vi "Write to Hardware.vi"(8 "error in":errorcluster, 9 "trigger values":dbl[](array[numeric]), 10 "Values in":dbl[](array[numeric]), 11 "Ballard ARINC-429 Tx Acyclic execution unit in":refnum<class "Tx Acyclic Labels Execution Unit.lvclass">) -> (0 "error out":errorcluster, 1 "trigger values out":dbl[](array[numeric]), 2 "Values out":dbl[](array[numeric]), 3 "Ballard ARINC-429 Tx Acyclic execution unit out":refnum<class "Tx Acyclic Labels Execution Unit.lvclass">)   [LabVIEW 2020, in "Ballard ARINC 429 Engine.lvlib" / "Implementation.lvlib" / "Tx Acyclic Labels Execution Unit.lvclass"]
uses:
  Tx Acyclic Labels Execution Unit.lvclass
  <instrlib>/BTI429Lib/BTI429LV.lvlib
  <instrlib>/BTI429Lib/Private/Tx/Data/Transmit Message Dynamic.vi
  Custom Device/Custom Device.lvlib
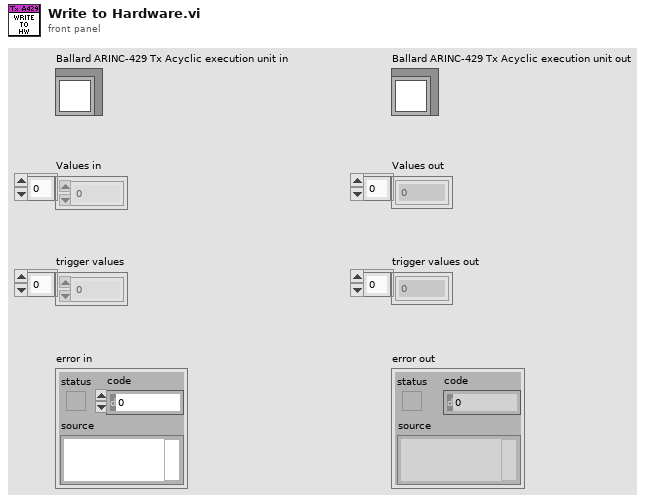
[diagram p1: front panel]
types:
  T1 = typedef "RT Hardware Channel Settings.ctl" = cluster{"channel #":u16, "channel handle":u64, "labels settings for RT":T2[]}
  T2 = typedef "RT Label Settings.ctl" = cluster{"Name":string, "xmlName":string, "label":T3, "transfer period":u32, "SDI_Enabled":bool, "SDI":u8, "parameter driver data":T4, "transfer type":T8, "has timestamp?":bool, "Label Disable/Trigger Channel Reference":T7, "Message Handle":u64, "Initialized?":bool, "Word Initial Raw Value":u32, "Label Timestamp Channel Data Reference":T9, "disabled":bool}
  T3 = typedef "Label.ctl" = u8
  T4 = typedef "RT Parameters.ctl" = cluster{"parameter definitions":T5[], "Tx parameter refs":T7[]}
  T5 = typedef "Parameter Definition.ctl" = cluster{"start index":i32, "size":i32, "encoding":T6, "signed":bool, "scale multiplier":dbl, "scale offset":dbl}
  T6 = typedef "Encoding and Decoding.lvlib/Encoding.ctl" = enum16{"BNR", "BCD", "Discrete"}
  T7 = typedef "Custom Device API.lvlib/Custom Device Item Ref.ctl" = u64
  T8 = typedef "Transfer Type.ctl" = enum16{"Scheduled", "Acyclic", "Block", "Strobe"}
  T9 = typedef "Custom Device API.lvlib/Data Reference.ctl" = i32
  T10 = typedef "Map of Values Indexes to Channel and Label Indexes.ctl" = map{i32, cluster{"channel index":i32, "label index":i32, "group values start index":i32, "values in group":i32}}
  T11 = cluster{"channel index":i32, "label index":i32, "group values start index":i32, "values in group":i32}
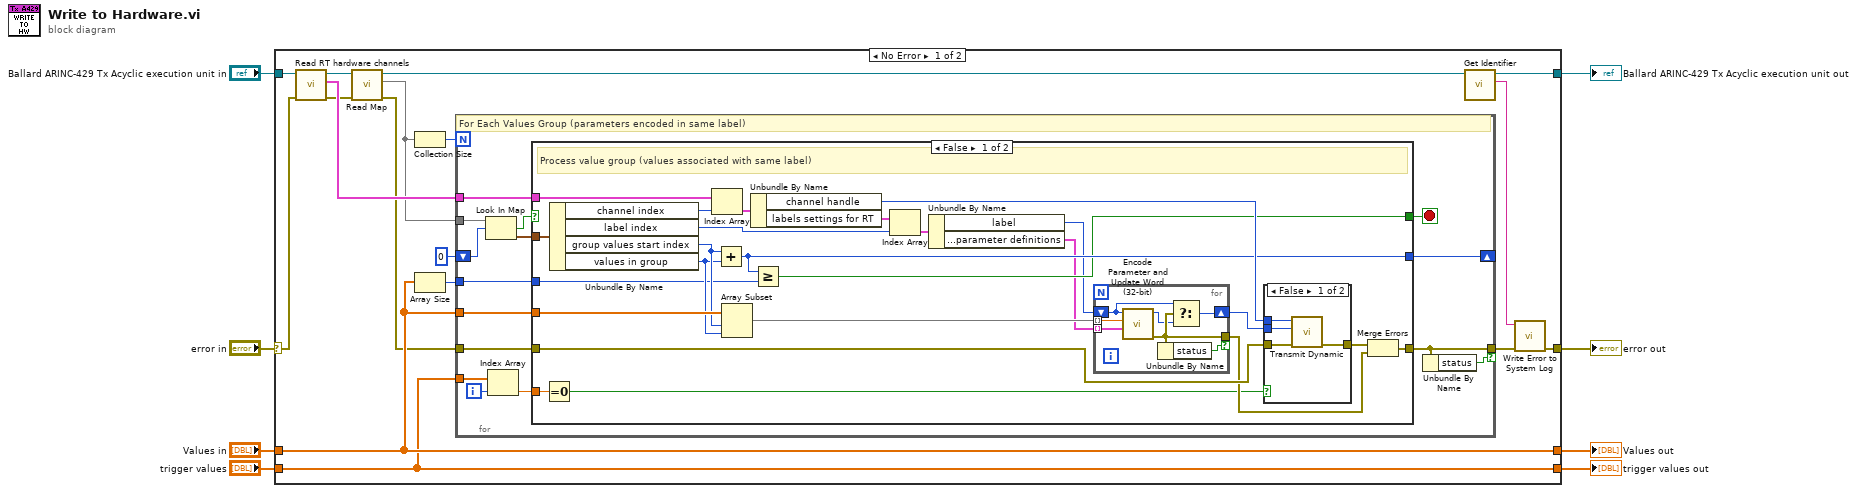
[diagram p0: block diagram]
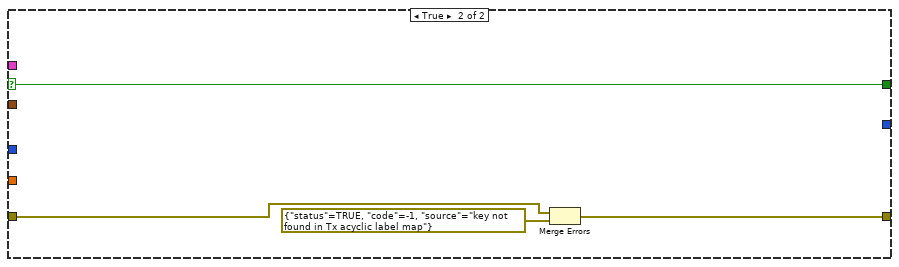
[diagram p3: hidden frame]
diagram:
  n1 = case shown="No Error" "error in" {
    selector: "error in" -> [w19 w83]
    tunnel: [w9 w83] -> w8
    tunnel: [w21 w82] -> w6
    tunnel: "Values in" -> [w21 w82]
    tunnel: [w12 w84] -> w4
    tunnel: "Ballard ARINC-429 Tx Acyclic execution unit in" -> [w18 w84]
    tunnel: "trigger values" -> [w14 w81]
    tunnel: [w14 w81] -> w1
    frame No Error {
      n2 = call "Read RT hardware channels.vi"("error in"=w19, "Ballard ARINC-429 Tx Acyclic execution unit in"=w18) -> ("error out"=w16:errorcluster, "RT hardware channels"=w25:T1[], "Ballard ARINC-429 Tx Acyclic execution unit out"=w17:refnum<class "Tx Acyclic Labels Execution Unit.lvclass">)  [unwired: 7 in]
      n3 = call "Read Map.vi"("error in"=w16, "Ballard ARINC-429 Tx Acyclic execution unit in"=w17) -> ("error out"=w15:errorcluster, "map from values indexes to RT info indexes"=w22:T10, "Ballard ARINC-429 Tx Acyclic execution unit out"=w13:refnum<class "Tx Acyclic Labels Execution Unit.lvclass">)  [unwired: 7 in]
      n4 = Collection Size(1:w22) -> (0:w23:i32)
      n5 = Array Size(array=w21) -> (size(s)=w20:i32)
      n6 = for {
        N: w23 -> [_]
        tunnel: w21 -> [w35]
        tunnel: w22 -> [w38]
        shift-right: [w34] -> _
        shift-left: 0 -> [w37]
        tunnel: w15 -> [w40]
        tunnel: [w30] -> w10 if=w29
        tunnel: w20 -> [w32]
        tunnel: w25 -> [w39]
        tunnel: w14 -> [w27]
        i -> [w28]
        stop <- w31 stop-if-true
        # "For Each Values Group (parameters encoded in same label)"
        n7 = Look In Map(map=w38, key=w37) -> (key not found?=w33:bool, value=w36:T11)  [unwired: 1 in]
        n8 = Index Array(array=w27, index=w28) -> (element=w26:dbl)
        n9 = case shown="False" w33 {
          selector: w33 -> [_ w77]
          tunnel: w40 -> [w49 w80]
          tunnel: [w48 w78] -> w30
          tunnel: w39 -> [w54 _]
          tunnel: w36 -> [w64 _]
          tunnel: w35 -> [w63 _]
          tunnel: [w52 _] -> w34
          tunnel: w32 -> [w51 _]
          tunnel: [w50 w77] -> w31
          tunnel: w26 -> [w47 _]
          frame False {
            # "Process value group (values associated with same label)"
            n10 = Equal To 0?(x=w47) -> (x = 0?=w41:bool)
            n11 = Unbundle By Name(w64) -> ("channel index"=w57:i32, "label index"=w58:i32, "group values start index"=w62:i32, "values in group"=w61:i32)
            n12 = Index Array(array=w54, index=w57) -> (element=w56:T1)
            n13 = Add(x=w62, y=w61) -> (x+y=w52:i32)
            n14 = Array Subset(array=w63, index=w62, length=w61) -> (w60:dbl[])
            n15 = Unbundle By Name(w56) -> ("channel handle"=w53:u64, "labels settings for RT"=w55:T2[])
            n16 = Greater Or Equal?(x=w52, y=w51) -> (x >= y?=w50:bool)
            n17 = Index Array(array=w55, index=w58) -> (element=w59:T2)
            n18 = Unbundle By Name(w59) -> ("label"=w45:T3, "parameter driver data.parameter definitions"=w46:T5[])
            n19 = for {
              tunnel: w60 -> [w76] mode=indexing
              shift-right: [w70] -> w44
              shift-left: w45 -> [w74]
              tunnel: w46 -> [w75] mode=indexing
              tunnel: [w73] -> w42 if=w72
              n20 = call "Encode Parameter and Update Word (32-bit).vi"("parameter definition"=w75, "parameter value"=w76, "word in"=w74) -> ("error out"=w73:errorcluster, "word out"=w71:u32)  [unwired: 7 in]
              n21 = Unbundle By Name(w73) -> ("status"=w72:bool)
              n22 = Select(t=w74, s=w73, f=w71) -> (s? t:f=w70:u32)
            }
            n23 = case shown="False" w41 {
              tunnel: w53 -> [w68 _]
              tunnel: w49 -> [w67 w69]
              tunnel: w44 -> [w66 _]
              tunnel: [w65 w69] -> w43
              frame False {
                n24 = call-poly <instrlib>:"Transmit Dynamic.vi"("error in (no error)"=w67, "message data"=w66, "channel handle in"=w68) -> ("error out"=w65:errorcluster)  [unwired: 7 in, 1 out]
              }
              frame True {
              }
            }
            n25 = Merge Errors(w43, w42) -> (w48:errorcluster)
          }
          frame True {
            n26 = Merge Errors(w80, errorcluster {"status"=TRUE, "code"=-1, "source"="key not found in Tx acyclic label map"} ("error in")) -> (w78:errorcluster)
          }
        }
        n27 = Unbundle By Name(w30) -> ("status"=w29:bool)
      }
      n28 = call-dynamic "Get Identifier.vi"("Ballard ARINC-429 Execution Unit in"=w13) -> ("identifier"=w11:string, "Ballard ARINC-429 Execution Unit out"=w12:refnum<class "Tx Acyclic Labels Execution Unit.lvclass">)  [unwired: 8 in, 1 out]
      n29 = call "Write Error to System Log.vi"("error in"=w10, "identifier"=w11) -> ("error out"=w9:errorcluster)  [unwired: 9 in]
    }
    frame Error {
    }
  }
  "error out" <- w8
  "Ballard ARINC-429 Tx Acyclic execution unit out" <- w4
  "Values out" <- w6
  "trigger values out" <- w1
